vi "Cursor2px.vi"(6 "micron/pixel":dbl=2.0, 9 "Image dimension":i32, 10 "Picturebox dimension":i32, 11 "Cursor dimension":i32) -> (1 "Cluster":cluster{dbl, dbl}, 3 "mm value":dbl)   [LabVIEW 2019]
doc: "Given cursor coordinates, picturebox dimensions, determine true mm value displacement from origin"
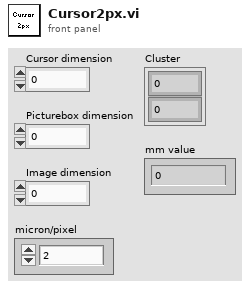
[diagram p1: front panel]
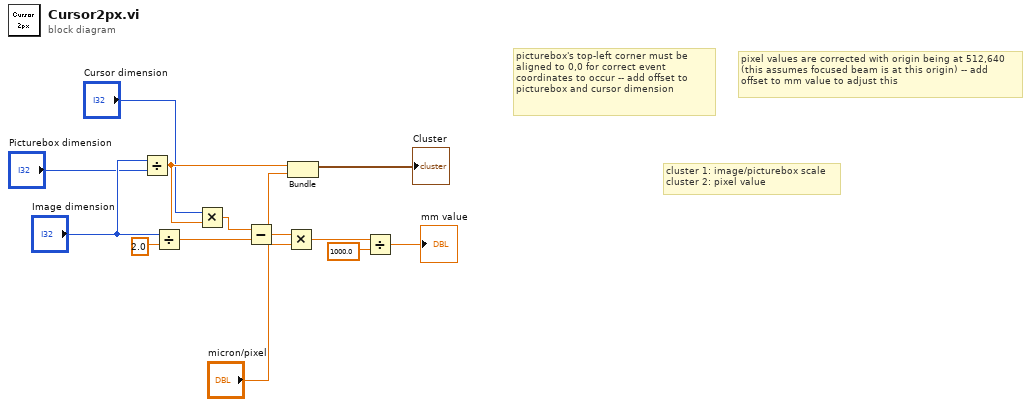
[diagram p0: block diagram]
diagram:
  # "cluster 1: image/picturebox scale\ncluster 2: pixel value"
  # "picturebox's top-left corner must be aligned to 0,0 for correct event coordinates to occur -- add offset to \npicturebox and cursor dimension"
  # "pixel values are corrected with origin being at 512,640\n(this assumes focused beam is at this origin) -- add \noffset to mm value to adjust this"
  n1 = Divide(x="Image dimension", y="Picturebox dimension") -> (x/y=w11:dbl)
  n2 = Divide(x="Image dimension", y=2.0) -> (x/y=w6:dbl)
  n3 = Multiply(x="Cursor dimension", y=w11) -> (x*y=w1:dbl)
  n4 = Subtract(x=w1, y=w6) -> (x-y=w12:dbl)
  n5 = Multiply(x=w12, y="micron/pixel") -> (x*y=w10:dbl)
  n6 = Bundle(w11, w12) -> (→"Cluster":cluster{dbl, dbl})  [unwired: 1 in]
  n7 = Divide(x=w10, y=1000.0) -> (x/y=→"mm value":dbl)
